vi "Practica6_MotorCC.vi"() -> ()   [LabVIEW 2015]
uses:
  <vilib>/LabVIEW Interface for Arduino/Type Defs/Pin Mode.ctl
  <vilib>/LabVIEW Interface for Arduino/LabVIEW Interface for Arduino.lvlib
panel:
  in  "stop":bool
  out "Derecha":bool
  out "Izquierda":bool
  in  "Velocidad y Sentido de Giro":i8(knob) scale=-100.0..100.0
  # "Gobierno de un Motor de CC \nAsigando Direccion y Velocidad"
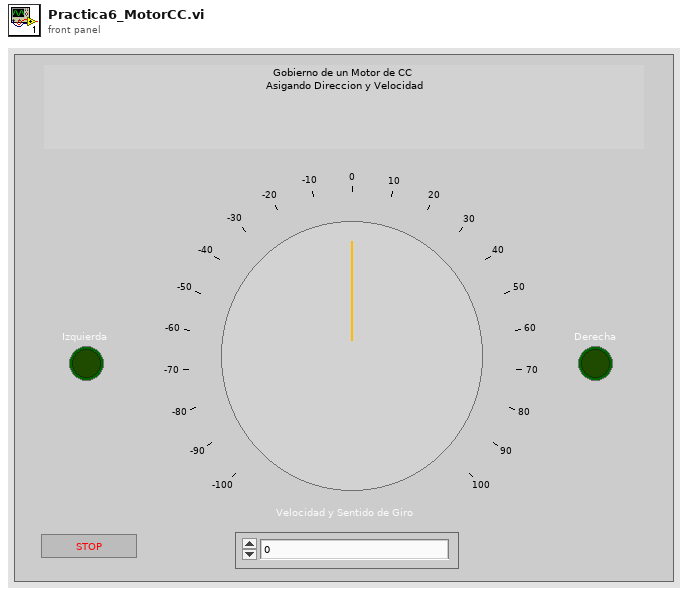
[diagram p1: front panel]
types:
  T1 = typedef "LabVIEW Interface for Arduino.lvlib/Pin Mode.ctl" = enum8{"Input", "Output"}
  T2 = typedef "LabVIEW Interface for Arduino.lvlib/Arduino Resource.ctl" = cluster{"VISA resource":refnum<visa-resource-name>, "Board Type":T3, "Connection Type":enum8{"USB / Serial"}, "Bytes Per Packet (15)":u8}
  T3 = typedef "LabVIEW Interface for Arduino.lvlib/Board Type.ctl" = enum16{"Uno", "Dimuelanove w/Atmega 328", "Mega 2560"}
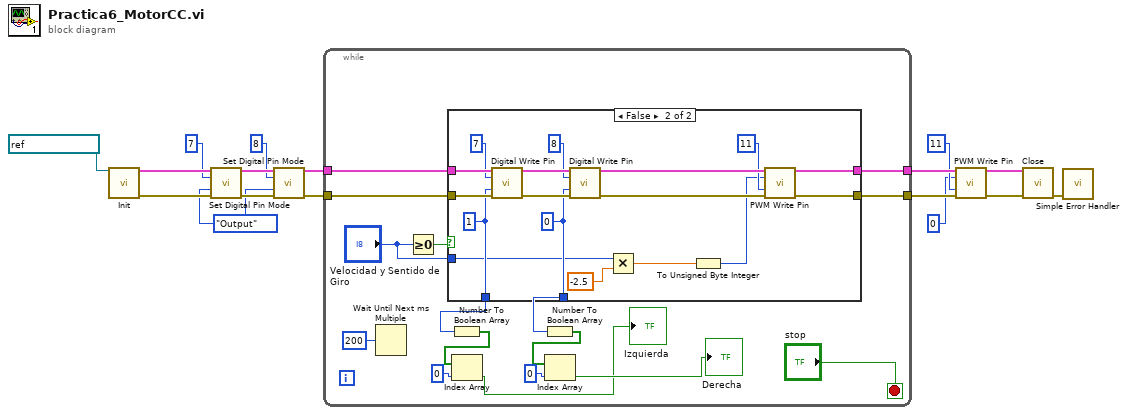
[diagram p0: block diagram]
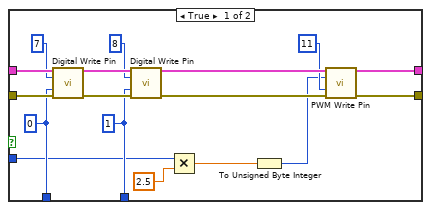
[diagram p2: hidden frame]
diagram:
  w12 = Pin_Mode."Output" ("Pin Mode (Input)")
  n1 = call <vilib>:"Init.vi"("VISA resource"=refnum<visa-resource-name> "COM3") -> ("Arduino Resource"=w16:T2, "error out"=w13:errorcluster)  [unwired: 17 in]
  n2 = call <vilib>:"Set Digital Pin Mode.vi"("Arduino Resource"=w16, "Digital I/O Pin"=u8 7, "Pin Mode (Input)"=w12, "error in"=w13) -> ("Arduino Resource"=w15:T2, "error out"=w14:errorcluster)  [unwired: 10 in]
  n3 = call <vilib>:"Set Digital Pin Mode.vi"("Arduino Resource"=w15, "Digital I/O Pin"=u8 8, "Pin Mode (Input)"=w12, "error in"=w14) -> ("Arduino Resource"=w9:T2, "error out"=w8:errorcluster)  [unwired: 10 in]
  n4 = while {
    tunnel: w9 -> [w33]
    tunnel: w8 -> [w32]
    tunnel: [w31] -> w7
    tunnel: [w30] -> w6
    stop <- "stop" stop-if-true
    n5 = Wait Until Next ms Multiple(millisecond multiple=u32 200) -> ()  [unwired: 1 out]
    n6 = Greater Or Equal To 0?(x="Velocidad y Sentido de Giro") -> (x >= 0?=w28:bool)
    n7 = case shown="False" w28 {
      tunnel: w33 -> [w50 w67]
      tunnel: w32 -> [w49 w66]
      tunnel: [w44 w61] -> w31
      tunnel: [w43 w60] -> w30
      tunnel: [w36 w53] -> w26
      tunnel: [w35 w52] -> w21
      tunnel: "Velocidad y Sentido de Giro" -> [w34 w51]
      frame True {
        w35 = u8 1 ("Value (0)")
        w36 = u8 0 ("Value (0)")
        n8 = call <vilib>:"Digital Write Pin.vi"("Arduino Resource"=w50, "Digital I/O Pin (0)"=u8 7, "Value (0)"=w36, "error in"=w49) -> ("Arduino Resource"=w47:T2, "error out"=w48:errorcluster)  [unwired: 10 in]
        n9 = call <vilib>:"Digital Write Pin.vi"("Arduino Resource"=w47, "Digital I/O Pin (0)"=u8 8, "Value (0)"=w35, "error in"=w48) -> ("Arduino Resource"=w46:T2, "error out"=w45:errorcluster)  [unwired: 10 in]
        n10 = Multiply(x=w34, y=2.5) -> (x*y=w39:dbl)
        n11 = To Unsigned Byte Integer(number=w39) -> (unsigned 8bit integer=w38:u8)
        n12 = call <vilib>:"PWM Write Pin.vi"("Arduino Resource"=w46, "Duty Cycle (0 - 255)"=w38, "PWM Pin (3)"=u8 11, "error in"=w45) -> ("Arduino Resource"=w43:T2, "error out"=w44:errorcluster)  [unwired: 10 in]
      }
      frame False {
        w52 = u8 0 ("Value (0)")
        w53 = u8 1 ("Value (0)")
        n13 = call <vilib>:"Digital Write Pin.vi"("Arduino Resource"=w67, "Digital I/O Pin (0)"=u8 7, "Value (0)"=w53, "error in"=w66) -> ("Arduino Resource"=w64:T2, "error out"=w65:errorcluster)  [unwired: 10 in]
        n14 = call <vilib>:"Digital Write Pin.vi"("Arduino Resource"=w64, "Digital I/O Pin (0)"=u8 8, "Value (0)"=w52, "error in"=w65) -> ("Arduino Resource"=w63:T2, "error out"=w62:errorcluster)  [unwired: 10 in]
        n15 = Multiply(x=w51, y=-2.5) -> (x*y=w56:dbl)
        n16 = To Unsigned Byte Integer(number=w56) -> (unsigned 8bit integer=w55:u8)
        n17 = call <vilib>:"PWM Write Pin.vi"("Arduino Resource"=w63, "Duty Cycle (0 - 255)"=w55, "PWM Pin (3)"=u8 11, "error in"=w62) -> ("Arduino Resource"=w60:T2, "error out"=w61:errorcluster)  [unwired: 10 in]
      }
    }
    n18 = Number To Boolean Array(number=w26) -> (Boolean array=w25:bool[])
    n19 = Index Array(array=w25, index=0) -> (element=→"Izquierda":bool)
    n20 = Number To Boolean Array(number=w21) -> (Boolean array=w24:bool[])
    n21 = Index Array(array=w24, index=0) -> (element=→"Derecha":bool)
  }
  n22 = call <vilib>:"PWM Write Pin.vi"("Arduino Resource"=w6, "Duty Cycle (0 - 255)"=u8 0, "PWM Pin (3)"=u8 11, "error in"=w7) -> ("Arduino Resource"=w5:T2, "error out"=w4:errorcluster)  [unwired: 10 in]
  n23 = call <vilib>:"Close.vi"("Arduino Resource"=w5, "error in"=w4) -> ("error out"=w1:errorcluster)  [unwired: 13 in]
  n24 = call <vilib>:"Simple Error Handler.vi"("error in (no error)"=w1) -> ()  [unwired: 4 in, 5 out]
